vi "Host_HealthCheck_Color.vi"(1 "In range?":bool) -> (0 "Color out":u32)   [LabVIEW 2018]
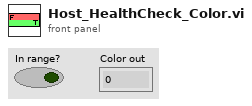
[diagram p1: front panel]
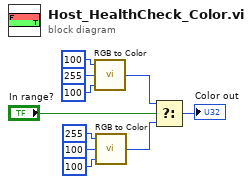
[diagram p0: block diagram]
diagram:
  n1 = call <vilib>:"RGB to Color.vi"("B"=u8 100, "G"=u8 255, "R"=u8 100) -> ("Color"=w1:u32)
  n2 = call <vilib>:"RGB to Color.vi"("B"=u8 100, "G"=u8 100, "R"=u8 255) -> ("Color"=w8:u32)
  n3 = Select(t=w1, s="In range?", f=w8) -> (s? t:f=→"Color out":u32)
